vi "act_4-conv_C_F.vi"() -> ()   [LabVIEW 2010]
panel:
  out "Deg F":dbl
  in  "Deg C":dbl
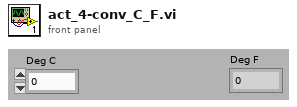
[diagram p1: front panel]
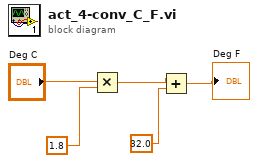
[diagram p0: block diagram]
diagram:
  n1 = Multiply(x="Deg C", y=1.8) -> (x*y=w4:dbl)
  n2 = Add(x=w4, y=32.0) -> (x+y=→"Deg F":dbl)
